vi "Split Strings around Split String.vi"(6 "Left/Right":T1(ring), 8 "error in (no error)":errorcluster, 9 "Split string":string, 11 "Filtered File Names in":string[](array[string])) -> (0 "error out":errorcluster, 1 "Residual Strings":string[](array[string]), 3 "Filtered File Names out":string[](array[string]))   [LabVIEW 2021, in "Strings.lvlib"]
uses:
  Strings.lvlib
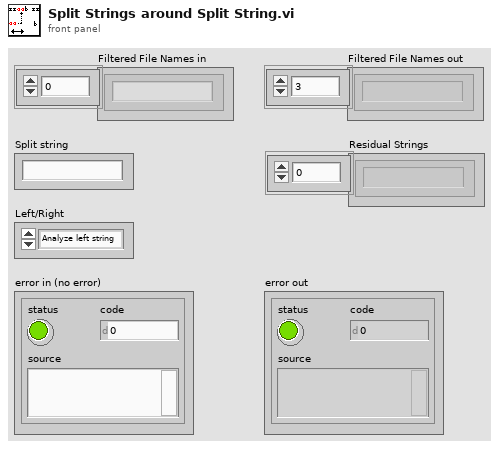
[diagram p1: front panel]
types:
  T1 = enum16{"Analyze left string", "Analyze right string"}
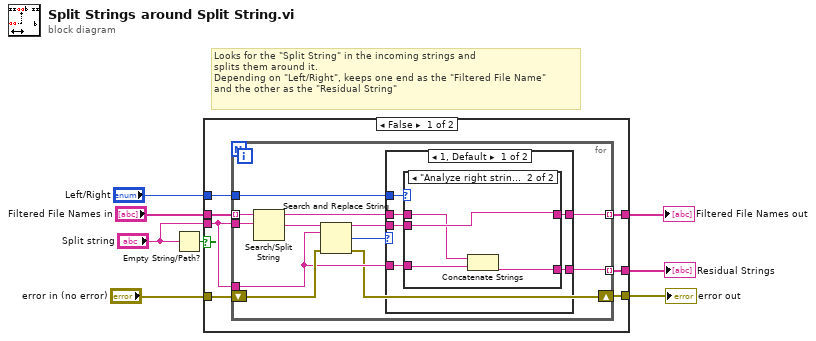
[diagram p0: block diagram]
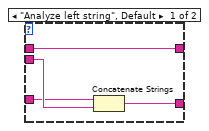
[diagram p2: hidden frame]
diagram:
  # "Looks for the \"Split String\" in the incoming strings and\nsplits them around it.\nDepending on \"Left/Right\", keeps one end as the \"Filtered File Name\"\nand the other as the \"Residual String\""
  n1 = Empty String/Path?(string/path="Split string") -> (empty?=w8:bool)
  n2 = case shown="False" w8 {
    tunnel: "Filtered File Names in" -> [w15 w44]
    tunnel: [w13 w44] -> w6
    tunnel: "error in (no error)" -> [w11 w43]
    tunnel: [w9 w43] -> w4
    tunnel: "Split string" -> [w12 _]
    tunnel: "Left/Right" -> [w14 _]
    tunnel: [w10 _] -> w1
    frame False {
      n3 = for {
        tunnel: w15 -> [w27] mode=indexing
        tunnel: w12 -> [w25]
        tunnel: w14 -> [w23]
        tunnel: [w20] -> w13 mode=indexing
        tunnel: w12 -> [w18]
        tunnel: [w19] -> w10 mode=indexing
        shift-right: [w16] -> w9
        shift-left: w11 -> [w24]
        n4 = Search/Split String(string=w27, search string/char (-)=w25) -> (substring before match=w21:string, match + rest of string=w26:string)  [unwired: 1 in, 1 out]
        n5 = Search and Replace String(input string=w26, search string=w18, error in=w24) -> (result string=w22:string, number of replacements=w17:i32, error out=w16:errorcluster)  [unwired: 5 in, 1 out]
        n6 = case shown="1, Default" w17 {
          tunnel: w23 -> [w33 _]
          tunnel: w22 -> [w32 _]
          tunnel: w21 -> [w31 w42]
          tunnel: [w30 w42] -> w20
          tunnel: [w29 _] -> w19
          tunnel: w18 -> [w28 _]
          frame 1, Default {
            n7 = case shown="\"Analyze right string\"" w33 {
              tunnel: w32 -> [w35 w41]
              tunnel: w31 -> [w37 w39]
              tunnel: [w37 w41] -> w30
              tunnel: [w36 w40] -> w29
              tunnel: w28 -> [w34 w38]
              frame "Analyze left string", Default {
                n8 = Concatenate Strings(w34, w35) -> (w36:string)
              }
              frame "Analyze right string" {
                n9 = Concatenate Strings(w39, w38) -> (w40:string)
              }
            }
          }
          frame 0 {
          }
        }
      }
    }
    frame True {
    }
  }
  "error out" <- w4
  "Filtered File Names out" <- w6
  "Residual Strings" <- w1
